vi "Add Error Message.vi"(7 "VI Ref":refnum<vi>, 10 "ErrorMessages":string, 11 "error in (no error)":errorcluster) -> (3 "error out":errorcluster)   [LabVIEW 2021]
doc: "用来收集错误的详细信息。例如数据库的连接字符串，打开数据库字符串。请将此模块添加到任何有可能出错的地方。\n2015-10-16 11:40:39\nBy：蒋松\nEmail：jiangsong@outlook.com\nSina: @sushu1051"
panel:
  out "source":string
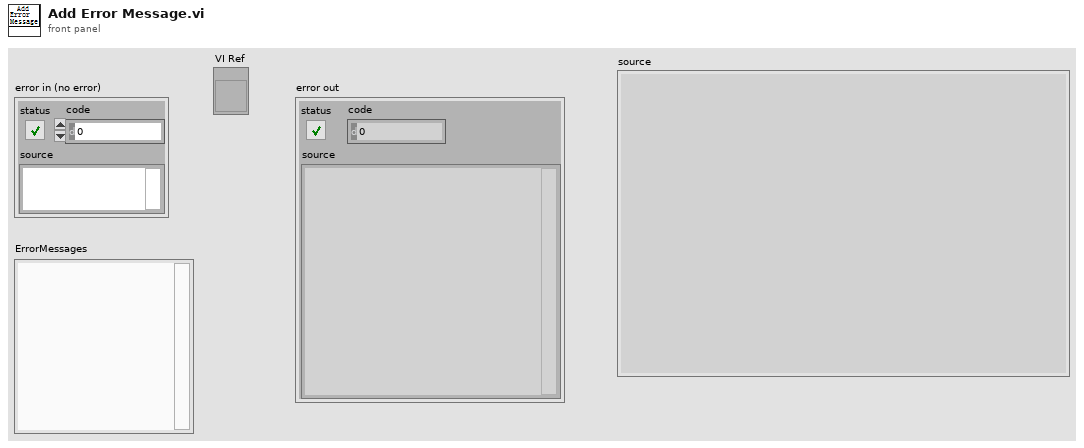
[diagram p1: front panel]
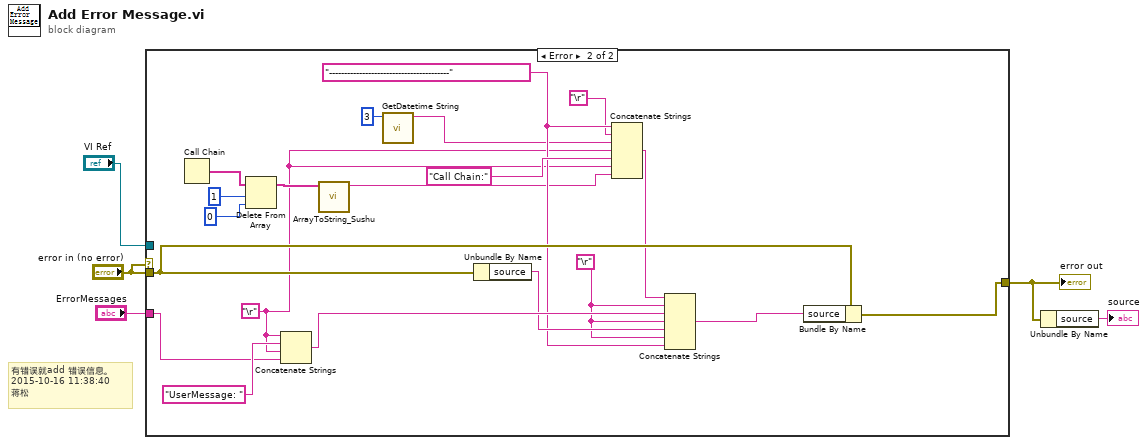
[diagram p0: block diagram]
diagram:
  # "有错误就add 错误信息。\n2015-10-16 11:38:40\n蒋松"
  n1 = case shown="Error" "error in (no error)" {
    tunnel: "ErrorMessages" -> [_ w20]
    tunnel: [w6 w18] -> w2
    tunnel: "error in (no error)" -> [w6 w25]
    tunnel: "VI Ref" -> [_ _]
    frame No Error {
    }
    frame Error {
      w16 = "----------------------------------------" ("string")
      w10 = "\r"
      w17 = "\r"
      n2 = Call Chain() -> (call chain=w15:string[])
      n3 = Delete From Array(array=w15, length=1, index=0) -> (array with subset deleted=w11:string[])  [unwired: 1 out]
      n4 = Concatenate Strings(w10, "UserMessage: " ("string"), w10, w20) -> (w23:string)
      n5 = call <userlib>:"ArrayToString_Sushu.vi"("Array"=w11) -> ("String"=w12:string)  [unwired: 10 in]
      n6 = call <userlib>:"GetDatetime String.vi"("u?"=3) -> ("date/time string"=w9:string)  [unwired: 5 in, 5 out]
      n7 = Unbundle By Name(w25) -> ("source"=w19:string)
      n8 = Concatenate Strings(w16, "\r", w9, w10, "Call Chain:" ("string"), w10, w12) -> (w22:string)
      n9 = Concatenate Strings(w22, w17, w23, w17, w19, w17, w16) -> (w26:string)
      n10 = Bundle By Name(cluster=w25, "source"=w26) -> (w18:errorcluster)
    }
  }
  "error out" <- w2
  n11 = Unbundle By Name(w2) -> ("source"=→"source":string)
